vi "Loop_HW.vi"() -> ()   [LabVIEW 2017, in "TemplateSensor.lvlib"]
uses:
  TemplateSensor.lvlib
  Global_HW_Data Out.vi
  Cluster_HW Status.ctl
  Globals/Global_STOP.vi
panel:
  out "Sensor Value":dbl
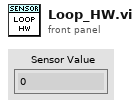
[diagram p1: front panel]
types:
  T1 = typedef "TemplateSensor.lvlib/Cluster_HW Status.ctl" = cluster{"Sensor Value":dbl}
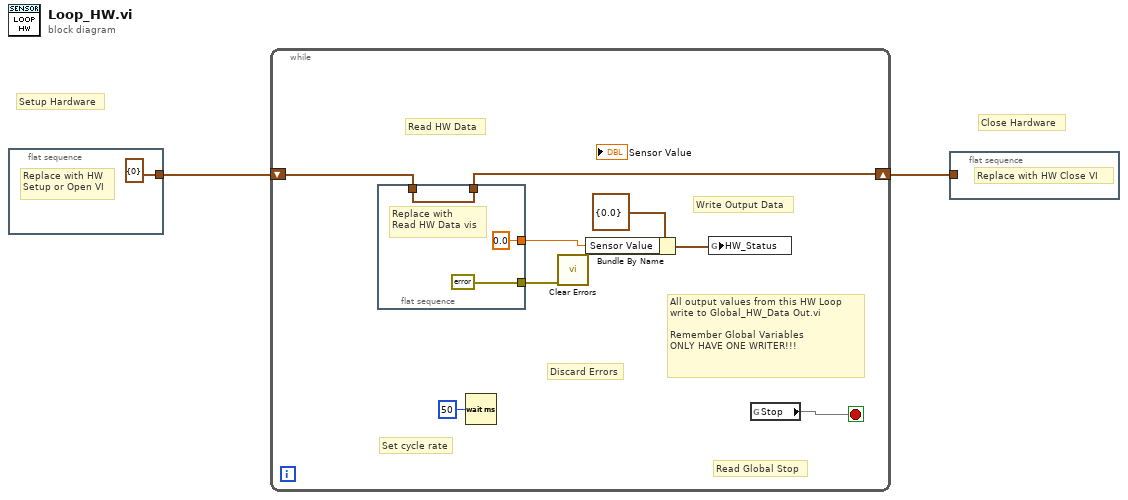
[diagram p0: block diagram]
diagram:
  # "Close Hardware"
  # "Setup Hardware"
  n1 = flat-sequence {
    tunnel: [cluster{i32} {0}] -> w2
    frame #0 {
      # "Replace with HW\nSetup or Open VI"
    }
  }
  n2 = while {
    shift-right: [w9] -> w1
    shift-left: w2 -> [w10]
    stop <- w4 stop-if-true
    # "Discard Errors"
    # "All output values from this HW Loop\nwrite to Global_HW_Data Out.vi\n\nRemember Global Variables\nONLY HAVE ONE WRITER!!!"
    # "Read HW Data"
    # "Read Global Stop"
    # "Set cycle rate"
    # "Write Output Data"
    n3 = flat-sequence {
      tunnel: w10 -> [w14]
      tunnel: [w14] -> w9
      tunnel: [errorcluster {"status"=FALSE, "code"=0, "source"=""} ("error constant")] -> w8
      tunnel: [0.0 ("Sensor Value")] -> w5
      frame #0 {
        # "Replace with\nRead HW Data vis"
      }
    }
    n4 = Wait (ms)(milliseconds to wait=u32 50) -> ()  [unwired: 1 out]
    n5 = call <vilib>:"Clear Errors.vi"("error in (no error)"=w8) -> ()  [unwired: 5 in, 2 out]
    n6 = Bundle By Name(cluster=T1 {"Sensor Value"=0.0} ("HW_Status"), "Sensor Value"=w5) -> (w6:T1)
    n7 = global write "Global_HW_Data Out.vi" "HW_Status"(w6) -> ()
    n8 = global read "Global_Stop.vi" "Stop"() -> (w4)
  }
  n9 = flat-sequence {
    tunnel: w1 -> [_]
    frame #0 {
      # "Replace with HW Close VI"
    }
  }
